vi "条件结构.vi"() -> ()   [LabVIEW 2017]
panel:
  out "字符串":string
  in  "布尔":bool
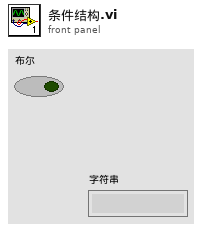
[diagram p1: front panel]
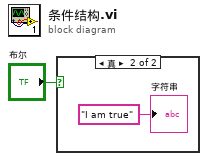
[diagram p0: block diagram]
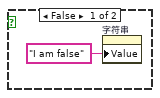
[diagram p2: hidden frame]
diagram:
  n1 = case shown="真" "布尔" {
    frame False {
      n2 = property on="字符串" class="Str"("Value"="I am false" ("字符串")) -> ()  [unwired: 2 in, 2 out]
    }
    frame True {
      "字符串" <- "I am true" ("字符串")
    }
  }
